vi "delme4.vi"   [LabVIEW 2020]
uses:
  Interop.MFilesAPI
types:
  T1 = cluster{"Name":string, "ViewType":i32, "Parent":i32, "ID":i32}[]
  T2 = cluster{"Name":string, "ViewType":i32, "Parent":i32, "ID":i32}
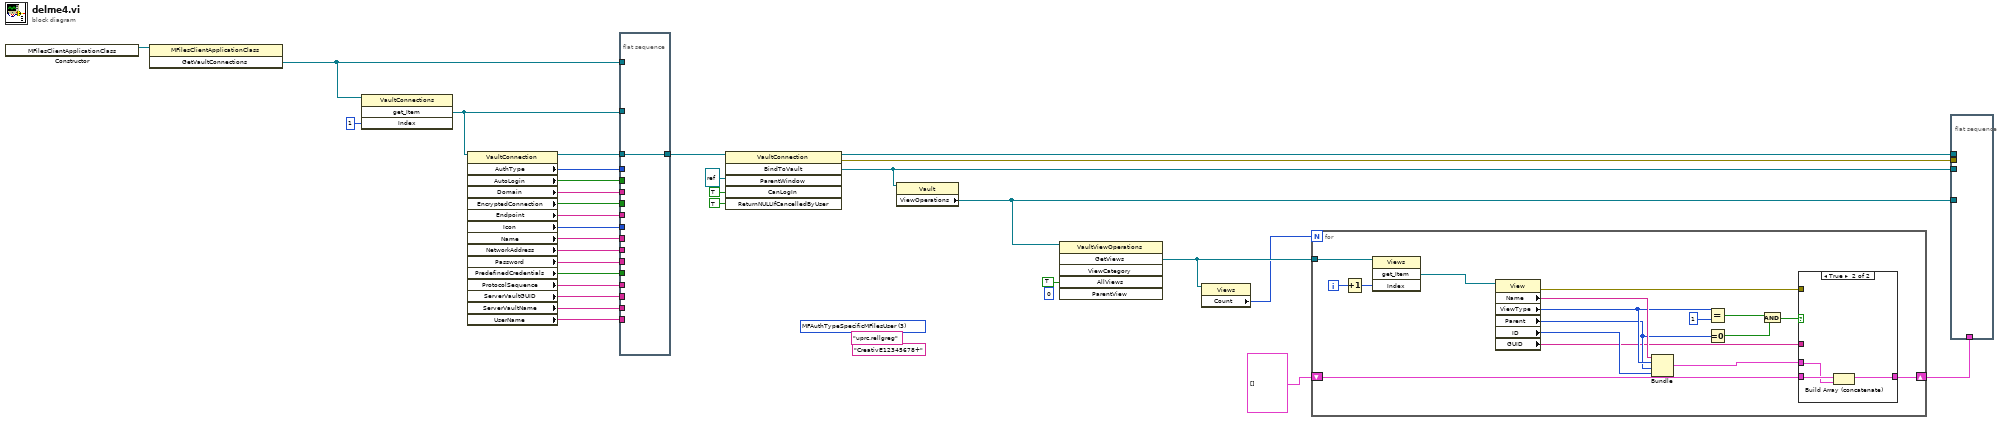
[diagram p0: block diagram]
diagram:
  (unwired) 0 ("ParentView")
  (unwired) 3 items=["MFAuthTypeUnknown", "MFAuthTypeLoggedOnWindowsUser", "MFAuthTypeSpecificWindowsUser", "MFAuthTypeSpecificMFilesUser"] ("AuthType")
  (unwired) "CreativE12345678+" ("Password")
  (unwired) "uprc.rellgreg" ("UserName")
  n1 = constructor class="MFilesClientApplicationClass"() -> (reference out=w11:refnum<k24>)  [unwired: 3 in, 2 out]
  n2 = invoke class="MFilesClientApplicationClass" method="GetVaultConnections"(reference=w11) -> ("GetVaultConnections"=w32:refnum<k24>)  [unwired: 2 in, 2 out]
  n3 = invoke class="VaultConnections" method="get_Item"(reference=w32, "Index"=1) -> ("get_Item"=w30:refnum<k24>)  [unwired: 2 in, 3 out]
  n4 = property class="VaultConnection"(reference=w30) -> (reference out=w15:refnum<k24>, "AuthType"=w29:i32, "AutoLogin"=w28:bool, "Domain"=w27:string, "EncryptedConnection"=w26:bool, "Endpoint"=w25:string, "Icon"=w24:u8[], "Name"=w23:string, "NetworkAddress"=w22:string, "Password"=w21:string, "PredefinedCredentials"=w20:bool, "ProtocolSequence"=w19:string, "ServerVaultGUID"=w18:string, "ServerVaultName"=w17:string, "UserName"=w16:string)  [unwired: 1 in, 1 out]
  n5 = flat-sequence {
    tunnel: w32 -> [_]
    tunnel: w30 -> [_]
    tunnel: w29 -> [_]
    tunnel: w28 -> [_]
    tunnel: w27 -> [_]
    tunnel: w26 -> [_]
    tunnel: w25 -> [_]
    tunnel: w24 -> [_]
    tunnel: w23 -> [_]
    tunnel: w22 -> [_]
    tunnel: w21 -> [_]
    tunnel: w20 -> [_]
    tunnel: w19 -> [_]
    tunnel: w18 -> [_]
    tunnel: w17 -> [_]
    tunnel: w16 -> [_]
    tunnel: w15 -> [w33]
    tunnel: [w33] -> w14
    frame #0 {
    }
  }
  n6 = invoke class="VaultConnection" method="BindToVault"(reference=w14, "ParentWindow"=refnum<k24> refnum, "CanLogIn"=TRUE, "ReturnNULLIfCancelledByUser"=TRUE) -> (reference out=w13:refnum<k24>, error out=w12:errorcluster, "BindToVault"=w7:refnum<k24>)  [unwired: 2 in, 3 out]
  n7 = property class="Vault"(reference=w7) -> ("ViewOperations"=w6:refnum<k24>)  [unwired: 1 in, 2 out]
  n8 = invoke class="VaultViewOperations" method="GetViews"(reference=w6, "AllViews"=TRUE) -> ("GetViews"=w5:refnum<k24>)  [unwired: 4 in, 5 out]
  n9 = property class="Views"(reference=w5) -> ("Count"=w4:i32)  [unwired: 1 in, 2 out]
  n10 = for {
    N: w4 -> [_]
    tunnel: w5 -> [w50]
    shift-right: [w37] -> w1
    shift-left: T1 [] -> [w39]
    i -> [w48]
    n11 = Increment(x=w48) -> (x+1=w47:i32)
    n12 = invoke class="Views" method="get_Item"(reference=w50, "Index"=w47) -> ("get_Item"=w49:refnum<k24>)  [unwired: 2 in, 3 out]
    n13 = property class="View"(reference=w49) -> (error out=w36:errorcluster, "Name"=w46:string, "ViewType"=w45:i32, "Parent"=w43:i32, "ID"=w35:i32, "GUID"=w34:string)  [unwired: 1 in, 1 out]
    n14 = Bundle("Name"=w46, "ViewType"=w45, "Parent"=w43, "ID"=w35) -> (w38:T2)  [unwired: 1 in]
    n15 = Equal?(x=w45, y=1) -> (x = y?=w42:bool)
    n16 = Equal To 0?(x=w43) -> (x = 0?=w41:bool)
    n17 = And(x=w42, y=w41) -> (x .and. y?=w40:bool)
    n18 = case shown="True" w40 {
      tunnel: w39 -> [w51 w54]
      tunnel: w38 -> [_ w53]
      tunnel: [w51 w52] -> w37
      tunnel: w36 -> [_ _]
      tunnel: w34 -> [_ _]
      frame False {
      }
      frame True {
        n19 = Build Array (concatenate)(w54, w53) -> (w52:T1)
      }
    }
  }
  n20 = flat-sequence {
    tunnel: w7 -> [_]
    tunnel: w13 -> [_]
    tunnel: w12 -> [_]
    tunnel: w6 -> [_]
    tunnel: w1 -> [_]
    frame #0 {
    }
  }
